vi "SDG60ConfModulationCarrier.vi"(0 "VISA resource name":refnum<visa-resource-name>="USB0::0xF4EC::0x1101::SDG6XEBC5R0119::INSTR", 2 "Channel (1:Channel 1)":i32(ring)=1 items=["Channel 1"=1, "Channel 2"=2], 11 "error in (no error)":errorcluster) -> (4 "VISA resource name out":refnum<visa-resource-name>, 15 "error out":errorcluster)   [LabVIEW 2018]
doc: "Selects the waveform shape, frequency, amplitude, offset, and phase for standard waveforms (including Sine, Square, Ramp, Pulse, DC and Arb).\n\nNotes: \nTo configure other parameters for pulse waveforms please run the Configure Pulse VI. \nTo configure noise waveform please run the Configure Noise VI.\nTo configure other parameters for arbitrary waveforms please run the Create Arbitrary Waveform. \nTo configure PRBS waveform please run the Configure PRBS Waveform VI."
panel:
  in  "Delay (s)":dbl=1.0 format="%#_16g"
  in  "Fall  time(s)":dbl=1.0 format="%#_16g"
  in  "Rise time (s)":dbl=1.0 format="%#_16g"
  in  "Duty Cycle (%)":dbl=100.0 format="%#_16g"
  in  "Offset (V)":dbl format="%#_16g"
  in  "Amplitude (V)":dbl=1.0 format="%#_16g"
  in  "Phase (degree)":dbl format="%#_16g"
  in  "Frequency (1 Hz)":dbl=1000.0 format="%#_16g"
  in  "Mod wave shape (0:Sine)":u16(ring) items=["Sine", "Square", "Ramp", "Arb", "Pulse"]
  # "Modulation will be turned on, as needed to be on to change\nsettings"
  # "Pulse not settable on scope, unsure if working\nThese settings will be ignored unless using pulse"
  # "Range: 0.001Hz-1 MHz\n11 digit precision"
  # "Min: 2ns"
  # "Min: 2ns"
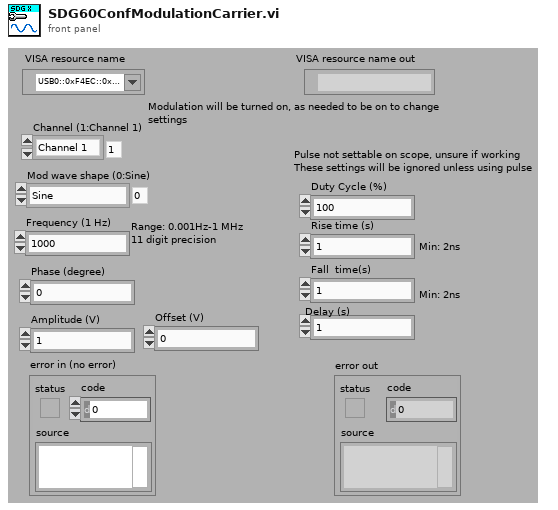
[diagram p1: front panel]
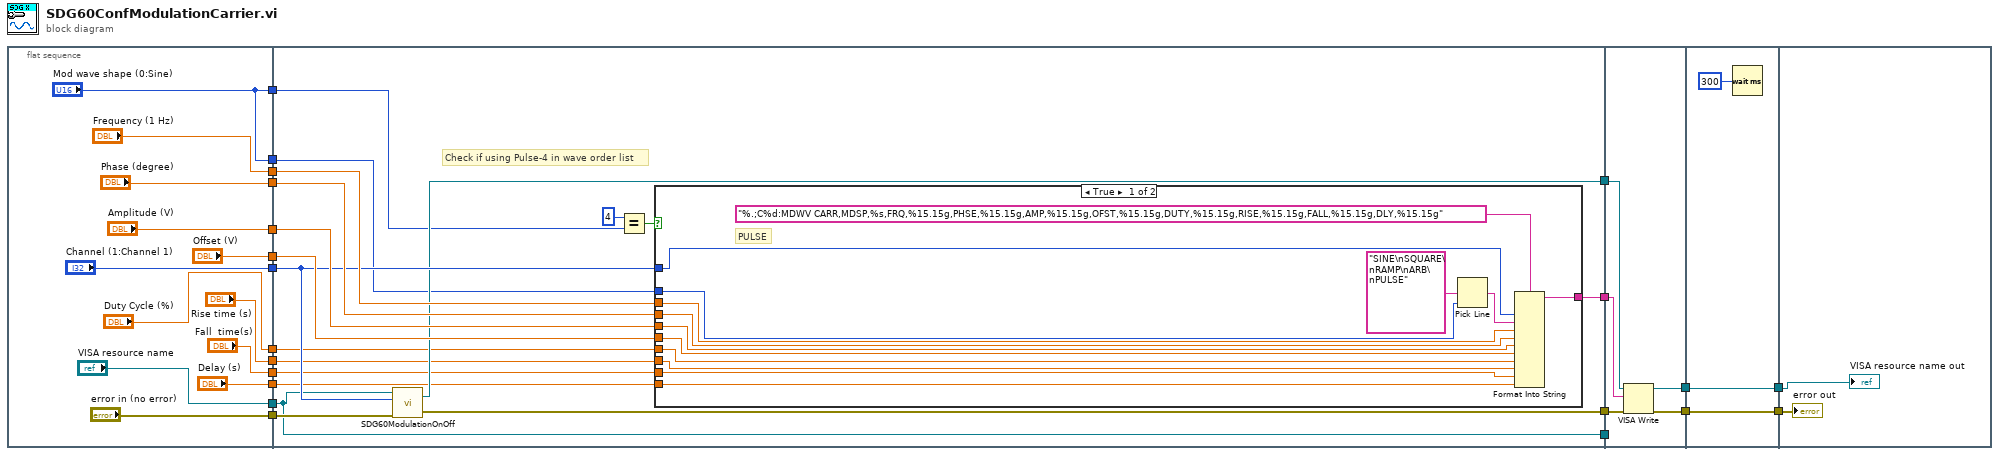
[diagram p0: block diagram]
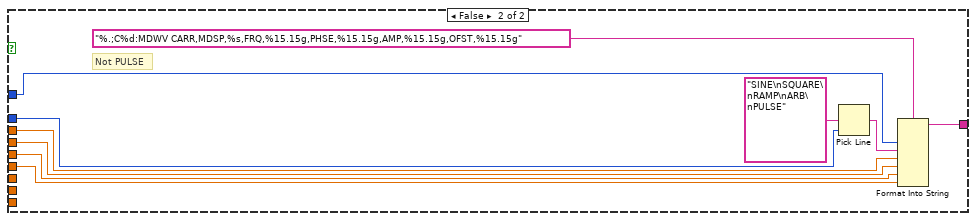
[diagram p2: hidden frame]
diagram:
  n1 = flat-sequence {
    tunnel: ["Mod wave shape (0:Sine)"] -> w21
    tunnel: ["Frequency (1 Hz)"] -> w20
    tunnel: ["Phase (degree)"] -> w19
    tunnel: ["Amplitude (V)"] -> w18
    tunnel: ["Channel (1:Channel 1)"] -> w17
    tunnel: ["Offset (V)"] -> w16
    tunnel: ["VISA resource name"] -> w15
    tunnel: ["error in (no error)"] -> w14
    tunnel: ["Duty Cycle (%)"] -> w7
    tunnel: ["Rise time (s)"] -> w6
    tunnel: ["Fall  time(s)"] -> w5
    tunnel: ["Delay (s)"] -> w4
    tunnel: ["Mod wave shape (0:Sine)"] -> w3
    tunnel: w21 -> [w41]
    tunnel: w20 -> [w51]
    tunnel: w19 -> [w50]
    tunnel: w18 -> [w49]
    tunnel: w17 -> [w46]
    tunnel: w16 -> [w48]
    tunnel: w15 -> [w45]
    tunnel: w14 -> [w47]
    tunnel: [w45] -> w13
    tunnel: [w44] -> w12
    tunnel: [w43] -> w11
    tunnel: [w42] -> w10
    tunnel: w7 -> [w37]
    tunnel: w6 -> [w36]
    tunnel: w5 -> [w35]
    tunnel: w4 -> [w34]
    tunnel: w3 -> [w38]
    tunnel: w13 -> [_]
    tunnel: w12 -> [w80]
    tunnel: w11 -> [w79]
    tunnel: w10 -> [w78]
    tunnel: [w77] -> w9
    tunnel: [w76] -> w8
    tunnel: w9 -> [w82]
    tunnel: w8 -> [w81]
    tunnel: [w82] -> w2
    tunnel: [w81] -> w1
    tunnel: w2 -> [w85]
    tunnel: w1 -> [w84]
    frame #0 {
    }
    frame #1 {
      # "Check if using Pulse-4 in wave order list"
      n2 = call "SDG60ModulationOnOff.vi"("error in (no error)"=w47, "Channel (1: Channel1)"=w46, "VISA resource name"=w45) -> ("error out"=w43:errorcluster, "VISA resource name out"=w42:refnum<visa-resource-name>)  [unwired: 1 in]
      n3 = Equal?(x=4, y=w38) -> (x = y?=w39:bool)
      n4 = case shown="True" w39 {
        tunnel: w51 -> [w62 w72]
        tunnel: w50 -> [w61 w71]
        tunnel: w49 -> [w60 w70]
        tunnel: w48 -> [w59 w69]
        tunnel: w46 -> [w58 w68]
        tunnel: [w57 w67] -> w44
        tunnel: w41 -> [w56 w66]
        tunnel: w37 -> [w55 _]
        tunnel: w36 -> [w54 _]
        tunnel: w35 -> [w53 _]
        tunnel: w34 -> [w52 _]
        frame True {
          # "PULSE"
          n5 = Pick Line(multi-line string="SINE\nSQUARE\nRAMP\nARB\nPULSE", line index=w56) -> (output string=w63:string)  [unwired: 1 in]
          n6 = Format Into String(format string="%.;C%d:MDWV CARR,MDSP,%s,FRQ,%15.15g,PHSE,%15.15g,AMP,%15.15g,OFST,%15.15g,DUTY,%15.15g,RISE,%15.15g,FALL,%15.15g,DLY,%15.15g", w58, w63, w62, w61, w60, w59, w55, w54, w53, w52) -> (resulting string=w57:string)  [unwired: 2 in, 1 out]
        }
        frame False {
          # "Not PULSE"
          n7 = Pick Line(multi-line string="SINE\nSQUARE\nRAMP\nARB\nPULSE", line index=w66) -> (output string=w73:string)  [unwired: 1 in]
          n8 = Format Into String(format string="%.;C%d:MDWV CARR,MDSP,%s,FRQ,%15.15g,PHSE,%15.15g,AMP,%15.15g,OFST,%15.15g", w68, w73, w72, w71, w70, w69) -> (resulting string=w67:string)  [unwired: 2 in, 1 out]
        }
      }
    }
    frame #2 {
      n9 = VISA Write(VISA resource name=w78, write buffer=w80, error in (no error)=w79) -> (VISA resource name out=w77:refnum<visa-resource-name>, error out=w76:errorcluster)  [unwired: 1 out]
    }
    frame #3 {
      n10 = Wait (ms)(milliseconds to wait=300) -> ()  [unwired: 1 out]
    }
    frame #4 {
      "error out" <- w84
      "VISA resource name out" <- w85
    }
  }
